vi "Avg Values 1.vi"(0 "Digital in":refnum<vi>, 1 "Numeric 8":dbl, 2 "Numeric 5":dbl, 3 "Numeric 9":dbl, 4 "Numeric 4":dbl, 6 "Numeric 6":dbl, 7 "Numeric 3":dbl, 8 "reference in":refnum<vi>, 9 "Numeric 12":dbl, 10 "Numeric 7":dbl, 11 "Numeric 11":dbl, 13 "Numeric 10":dbl) -> (14 "Numeric":dbl, 15 "Numeric 2":dbl)   [LabVIEW 2014]
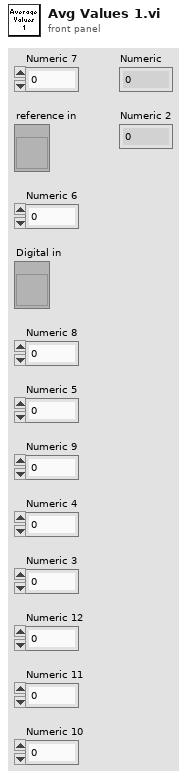
[diagram p1: front panel]
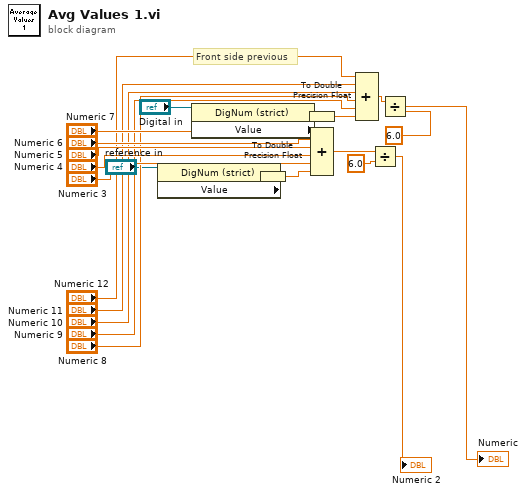
[diagram p0: block diagram]
diagram:
  # "Front side previous"
  n1 = property class="DigNum (strict)"(reference="reference in") -> ("Value"=w3:fxp<+,32,8>)  [unwired: 1 in, 2 out]
  n2 = property class="DigNum (strict)"(reference="Digital in") -> ("Value"=w4:fxp<+,64,16>)  [unwired: 1 in, 2 out]
  n3 = To Double Precision Float(number=w3) -> (double precision float=w20:dbl)
  n4 = To Double Precision Float(number=w4) -> (double precision float=w14:dbl)
  n5 = Compound Arithmetic op=ADD("Numeric 7", "Numeric 6", "Numeric 5", "Numeric 4", "Numeric 3", w20) -> (w13:dbl)
  n6 = Compound Arithmetic op=ADD("Numeric 12", "Numeric 11", "Numeric 10", "Numeric 8", "Numeric 9", w14) -> (w10:dbl)
  n7 = Divide(x=w13, y=6.0) -> (x/y=→"Numeric 2":dbl)
  n8 = Divide(x=w10, y=6.0) -> (x/y=→"Numeric":dbl)
